vi "HostTimeIndicators (1).vi"(11 "Array":i64[](array[numeric])) -> (0 "End Coast Time":dbl, 1 "End Push Time":dbl, 2 "Start Push Time":dbl, 3 "Current Time":dbl)   [LabVIEW 2017]
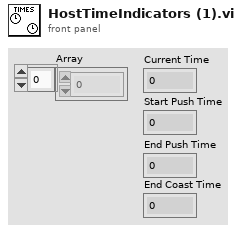
[diagram p1: front panel]
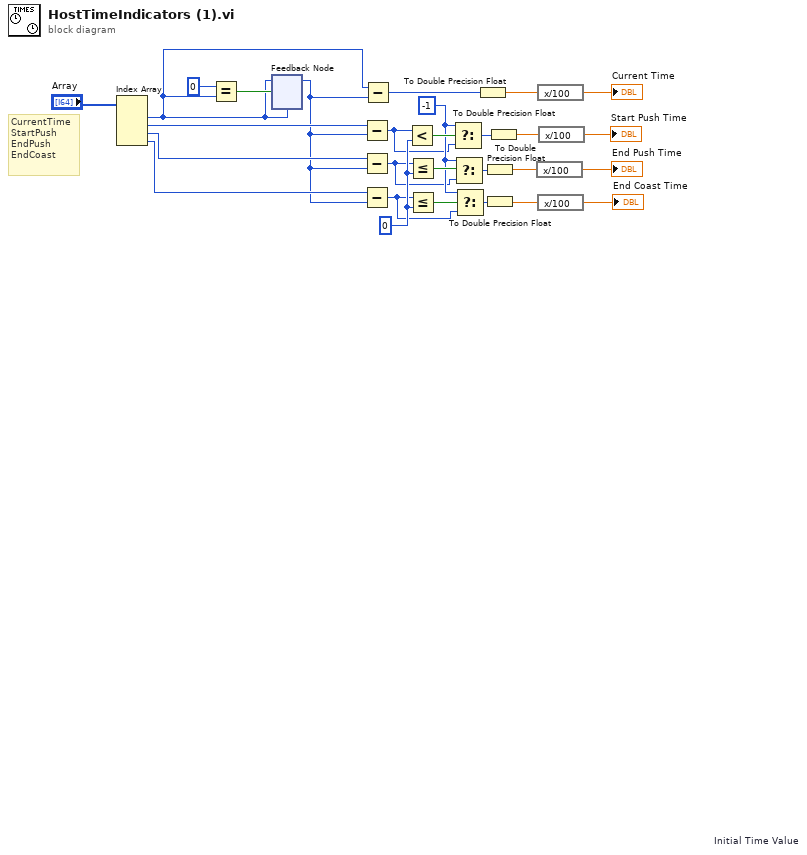
[diagram p0: block diagram]
diagram:
  w18 = i64 -1 ("y")
  w22 = i64 0 ("y")
  # "CurrentTime\nStartPush\nEndPush\nEndCoast"
  n1 = Index Array(array="Array") -> (element #1=w10:i64, element #2=w25:i64, element #3=w24:i64, element #4=w23:i64)  [unwired: 4 in]
  n2 = Equal?(x=i64 0, y=w10) -> (x = y?=w26:bool)
  n3 = feedback-in #1(w10, w26) -> ()
  n4 = feedback #1 "Initial Time Value"(w10) -> (w11:i64)
  n5 = Subtract(x=w25, y=w11) -> (x-y=w12:i64)
  n6 = Subtract(x=w24, y=w11) -> (x-y=w17:i64)
  n7 = Subtract(x=w23, y=w11) -> (x-y=w16:i64)
  n8 = Subtract(x=w10, y=w11) -> (x-y=w9:i64)
  n9 = Less?(x=w12, y=w22) -> (x < y?=w21:bool)
  n10 = Less Or Equal?(x=w17, y=w22) -> (x <= y?=w20:bool)
  n11 = Less Or Equal?(x=w16, y=w22) -> (x <= y?=w19:bool)
  n12 = Select(t=w18, s=w21, f=w12) -> (s? t:f=w15:i64)
  n13 = Select(t=w18, s=w20, f=w17) -> (s? t:f=w14:i64)
  n14 = Select(t=w18, s=w19, f=w16) -> (s? t:f=w13:i64)
  n15 = To Double Precision Float(number=w9) -> (double precision float=w8:dbl)
  n16 = To Double Precision Float(number=w14) -> (double precision float=w6:dbl)
  n17 = To Double Precision Float(number=w13) -> (double precision float=w5:dbl)
  n18 = To Double Precision Float(number=w15) -> (double precision float=w7:dbl)
  n19 = expression code="x/100"(w6) -> (→"End Push Time":dbl)
  n20 = expression code="x/100"(w8) -> (→"Current Time":dbl)
  n21 = expression code="x/100"(w5) -> (→"End Coast Time":dbl)
  n22 = expression code="x/100"(w7) -> (→"Start Push Time":dbl)
